vi "经纬转换－定位判断.vi"(10 "收到的字节":string) -> (2 "纬度":string, 3 "经度":string)   [LabVIEW 2018]
panel:
  out "纬度 2":string
  out "经度 2":string
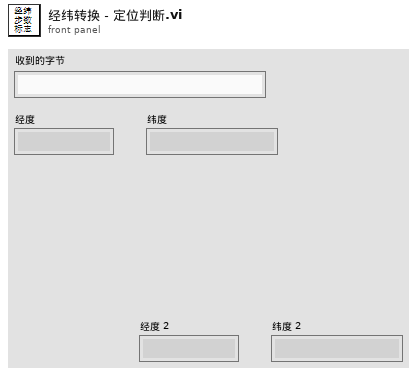
[diagram p1: front panel]
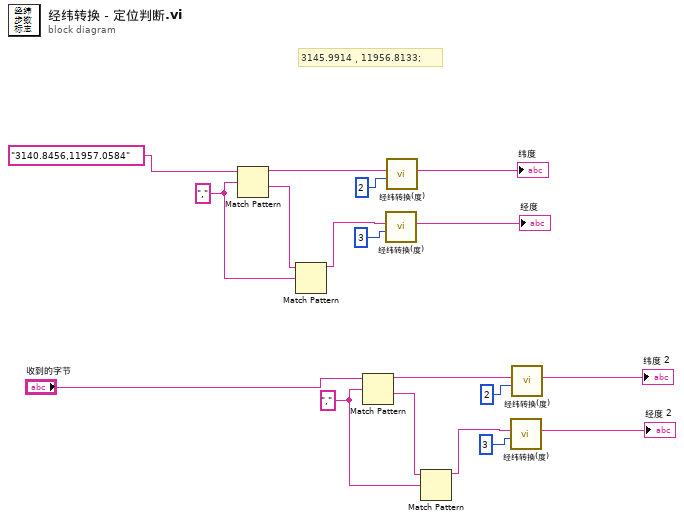
[diagram p0: block diagram]
diagram:
  w9 = "," ("正则表达式")
  w11 = "," ("正则表达式")
  # "3145.9914，11956.8133;"
  n1 = Match Pattern(string="3140.8456,11957.0584" ("收到的字节 2"), regular expression=w11) -> (before substring=w16:string, after substring=w13:string)  [unwired: 1 in, 2 out]
  n2 = Match Pattern(string=w13, regular expression=w11) -> (before substring=w12:string)  [unwired: 1 in, 3 out]
  n3 = Match Pattern(string="收到的字节", regular expression=w9) -> (before substring=w4:string, after substring=w7:string)  [unwired: 1 in, 2 out]
  n4 = call "经纬转换(度).vi"("整数部分长度"=3 ("长度（剩余）"), "经纬（度-分）"=w12) -> ("经纬（度）"=→"经度":string)  [unwired: 8 in, 1 out]
  n5 = call "经纬转换(度).vi"("整数部分长度"=2 ("长度（剩余）"), "经纬（度-分）"=w16) -> ("经纬（度）"=→"纬度":string)  [unwired: 8 in, 1 out]
  n6 = Match Pattern(string=w7, regular expression=w9) -> (before substring=w8:string)  [unwired: 1 in, 3 out]
  n7 = call "经纬转换(度).vi"("整数部分长度"=3 ("长度（剩余）"), "经纬（度-分）"=w8) -> ("经纬（度）"=→"经度 2":string)  [unwired: 8 in, 1 out]
  n8 = call "经纬转换(度).vi"("整数部分长度"=2 ("长度（剩余）"), "经纬（度-分）"=w4) -> ("经纬（度）"=→"纬度 2":string)  [unwired: 8 in, 1 out]
